vi "Get Old Class Version.vi"(10 "Numeric Value For LV Class":dbl, 11 "LV Class File Path":string="ModifiedClass.lvclass") -> (0 "error out":errorcluster, 2 "LV Class Version":string, 3 "ModifiedClass.lvclass":refnum<class "ModifiedClass.lvclass">)   [LabVIEW 2013]
uses:
  ModifiedClass.lvclass
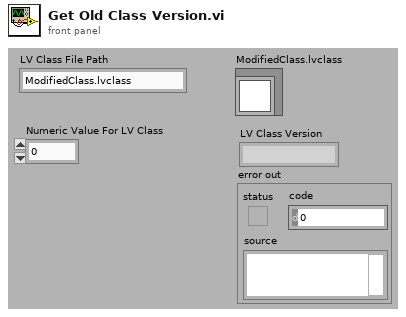
[diagram p1: front panel]
types:
  T1 = cluster{"Major":u16, "Minor":u16, "Fix":u16, "Build":u16}
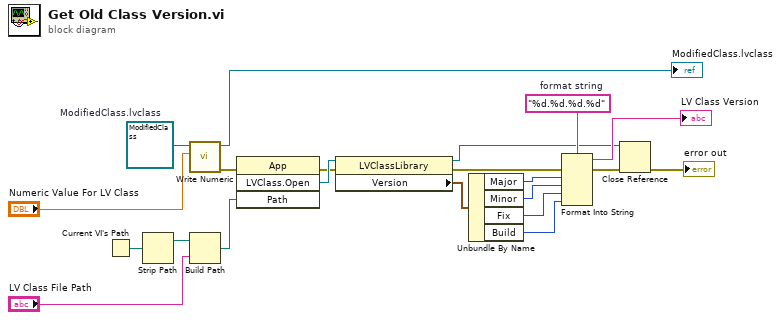
[diagram p0: block diagram]
diagram:
  w10 = "%d.%d.%d.%d"  # format string
  w4 = refnum<class "ModifiedClass.lvclass"> refnum  # ModifiedClass.lvclass
  n1 = Current VI's Path() -> (path=w21:path)
  n2 = Strip Path(path=w21) -> (stripped path=w20:path)  [unwired: 1 out]
  n3 = call-dynamic "Write Numeric.vi"("Numeric"="Numeric Value For LV Class", "ModifiedClass in"=w4) -> ("error out"=w2:errorcluster, "ModifiedClass out"=→"ModifiedClass.lvclass":refnum<class "ModifiedClass.lvclass">)  [unwired: 8 in]
  n4 = Build Path(base path=w20, name or relative path="LV Class File Path") -> (appended path=w18:path)
  n5 = invoke class="App" method="LVClass.Open"(error in=w2, "Path"=w18) -> (error out=w16:errorcluster, "LVClass.Open"=w17:refnum<vi>)  [unwired: 2 in, 2 out]
  n6 = property class="LVClassLibrary"(reference=w17, error in=w16) -> (reference out=w6:refnum<vi>, error out=w9:errorcluster, "Version"=w15:T1)
  n7 = Unbundle By Name(w15) -> ("Major"=w14:u16, "Minor"=w13:u16, "Fix"=w12:u16, "Build"=w11:u16)
  n8 = Format Into String(format string=w10, error in=w9, w14, w13, w12, w11) -> (resulting string=→"LV Class Version":string, error out=w7:errorcluster)  [unwired: 1 in]
  n9 = Close Reference(reference=w6, error in (no error)=w7) -> (error out=→"error out":errorcluster)
